vi "100kHz PID - nonPipelined.vi"() -> ()   [LabVIEW 2010]
uses:
  <vilib>/eio/EIONode/EIONode.xnode
  <vilib>/rvi/eio/nirviEIOImplementation/nirviEIOImplementation.xnode
  <vilib>/rvi/eio/common/nirviEmuClasses.ctl
  <vilib>/addons/control/pid/fpga.llb/XNode/niFpgaPID.xnode
  <vilib>/rvi/eio/common/nirviEmuTemplateMethod_noerrors.vi
panel:
  in  "PID.Setpoint.PID 2":i16
  in  "PID.Proportional Gain.PID 2":i16=1
  in  "PID.Integral Gain.PID 2":i16
  in  "PID.Derivative Gain.PID 2":i16
  in  "PID.Setpoint.PID 3":i16
  in  "PID.Proportional Gain.PID 3":i16=1
  in  "PID.Integral Gain.PID 3":i16
  in  "PID.Derivative Gain.PID 3":i16
  out "PID.Num Ticks":u32
  in  "PID.Setpoint.PID 1":i16
  in  "PID.Proportional Gain.PID 1":i16=1
  in  "PID.Integral Gain.PID 1":i16
  in  "PID.Derivative Gain.PID 1":i16
  in  "PID.Setpoint.PID 0":i16
  in  "PID.Proportional Gain.PID 0":i16=1
  in  "PID.Integral Gain.PID 0":i16
  in  "PID.Derivative Gain.PID 0":i16
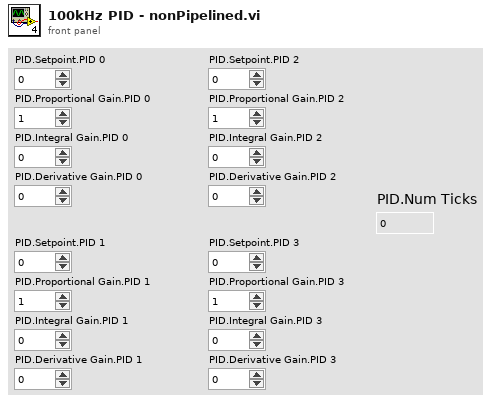
[diagram p1: front panel]
types:
  T1 = cluster{"proportional gain (Kc)":i16, "integral gain (Kc*Ts/Ti)":i16, "derivative gain (Kc*Td/Ts)":i16}
  T2 = typedef "nirviEmuClasses.ctl" = enum16{"IO Read", "IO Write", "Method", "Property Read", "Property Write"}
  T3 = cluster{"proportional gain (Kc)":fxp<+/-,16,8>, "proportional gain (Kc)":fxp<+/-,16,8>, "proportional gain (Kc)":fxp<+/-,16,8>}
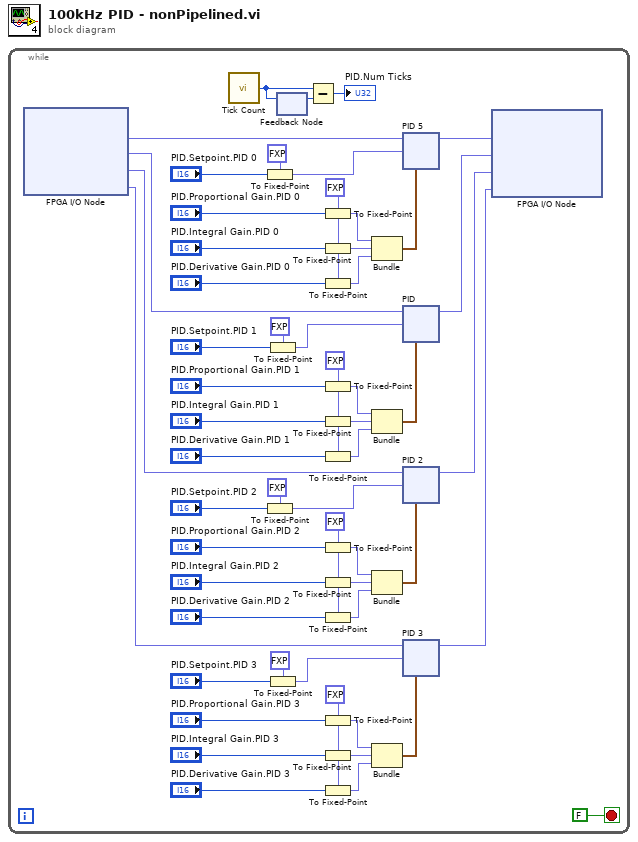
[diagram p0: block diagram]
diagram:
  n1 = while {
    stop <- FALSE stop-if-true
    w19 = fxp<+/-,16,8> 0.0 ("proportional gain (Kc)")
    w12 = fxp<+/-,16,8> 0.0 ("proportional gain (Kc)")
    w36 = fxp<+/-,16,8> 0.0 ("proportional gain (Kc)")
    w48 = fxp<+/-,16,8> 0.0 ("proportional gain (Kc)")
    n2 = xnode "FPGA I/O Node"() -> ("NI 9215/AI0"=w56:fxp<+/-,20,5>, "NI 9215/AI1"=w27:fxp<+/-,20,5>, "NI 9215/AI2"=w3:fxp<+/-,20,5>, "NI 9215/AI3"=w4:fxp<+/-,20,5>)  [unwired: 4 in, 4 out]
    n3 = call "Tick Count"() -> ("Tick Count(Ticks)"=w41:u32)
    n4 = To Fixed-Point(fixed-point type=fxp<+/-,16,5> 0.0 ("setpoint"), number="PID.Setpoint.PID 0") -> (fixed-point=w44:fxp<+/-,16,5>)
    n5 = To Fixed-Point(fixed-point type=fxp<+/-,16,5> 0.0 ("setpoint"), number="PID.Setpoint.PID 2") -> (fixed-point=w15:fxp<+/-,16,5>)
    n6 = To Fixed-Point(fixed-point type=fxp<+/-,16,5> 0.0 ("setpoint"), number="PID.Setpoint.PID 1") -> (fixed-point=w38:fxp<+/-,16,5>)
    n7 = To Fixed-Point(fixed-point type=fxp<+/-,16,5> 0.0 ("setpoint"), number="PID.Setpoint.PID 3") -> (fixed-point=w17:fxp<+/-,16,5>)
    n8 = feedback #1() -> (w42:u32)  [unwired: 1 in]
    n9 = feedback-in #1(w41) -> ()
    n10 = Subtract(x=w41, y=w42) -> (x-y=→"PID.Num Ticks":u32)
    n11 = To Fixed-Point(fixed-point type=w48, number="PID.Proportional Gain.PID 0") -> (fixed-point=w51:fxp<+/-,16,8>)
    n12 = To Fixed-Point(fixed-point type=w48, number="PID.Integral Gain.PID 0") -> (fixed-point=w50:fxp<+/-,16,8>)
    n13 = To Fixed-Point(fixed-point type=w48, number="PID.Derivative Gain.PID 0") -> (fixed-point=w49:fxp<+/-,16,8>)
    n14 = To Fixed-Point(fixed-point type=w36, number="PID.Proportional Gain.PID 1") -> (fixed-point=w33:fxp<+/-,16,8>)
    n15 = To Fixed-Point(fixed-point type=w36, number="PID.Integral Gain.PID 1") -> (fixed-point=w34:fxp<+/-,16,8>)
    n16 = To Fixed-Point(fixed-point type=w36, number="PID.Derivative Gain.PID 1") -> (fixed-point=w35:fxp<+/-,16,8>)
    n17 = To Fixed-Point(fixed-point type=w12, number="PID.Proportional Gain.PID 2") -> (fixed-point=w9:fxp<+/-,16,8>)
    n18 = To Fixed-Point(fixed-point type=w12, number="PID.Integral Gain.PID 2") -> (fixed-point=w10:fxp<+/-,16,8>)
    n19 = To Fixed-Point(fixed-point type=w12, number="PID.Derivative Gain.PID 2") -> (fixed-point=w11:fxp<+/-,16,8>)
    n20 = To Fixed-Point(fixed-point type=w19, number="PID.Proportional Gain.PID 3") -> (fixed-point=w22:fxp<+/-,16,8>)
    n21 = To Fixed-Point(fixed-point type=w19, number="PID.Integral Gain.PID 3") -> (fixed-point=w21:fxp<+/-,16,8>)
    n22 = To Fixed-Point(fixed-point type=w19, number="PID.Derivative Gain.PID 3") -> (fixed-point=w20:fxp<+/-,16,8>)
    n23 = Bundle("proportional gain (Kc)"=w51, "proportional gain (Kc)"=w50, "proportional gain (Kc)"=w49) -> (w52:T3)  [unwired: 1 in]
    n24 = Bundle("proportional gain (Kc)"=w33, "proportional gain (Kc)"=w34, "proportional gain (Kc)"=w35) -> (w32:T3)  [unwired: 1 in]
    n25 = Bundle("proportional gain (Kc)"=w9, "proportional gain (Kc)"=w10, "proportional gain (Kc)"=w11) -> (w8:T3)  [unwired: 1 in]
    n26 = Bundle("proportional gain (Kc)"=w22, "proportional gain (Kc)"=w21, "proportional gain (Kc)"=w20) -> (w23:T3)  [unwired: 1 in]
    n27 = xnode ("PID 5")("process variable"=w56, "setpoint"=w44, "PID gains"=w52) -> ("output"=w43:fxp<+/-,16,5>)  [unwired: 2 in]
    n28 = xnode ("PID")("process variable"=w27, "setpoint"=w38, "PID gains"=w32) -> ("output"=w28:fxp<+/-,16,5>)  [unwired: 2 in]
    n29 = xnode ("PID 2")("process variable"=w3, "setpoint"=w15, "PID gains"=w8) -> ("output"=w1:fxp<+/-,16,5>)  [unwired: 2 in]
    n30 = xnode ("PID 3")("process variable"=w4, "setpoint"=w17, "PID gains"=w23) -> ("output"=w2:fxp<+/-,16,5>)  [unwired: 2 in]
    n31 = xnode "FPGA I/O Node"("NI 9263/AO0"=w43, "NI 9263/AO1"=w28, "NI 9263/AO2"=w1, "NI 9263/AO3"=w2) -> ()  [unwired: 4 in, 4 out]
  }
